vi "Get Default Trigger.vi"(7 "Trigger Direction":T2, 8 "error in (no error)":errorcluster, 11 "Item Ref in":T3 format="%.0x") -> (0 "error out":errorcluster, 2 "Default Trigger":T1, 3 "Item Ref out":T3 format="%.0x")   [LabVIEW 2015, in "Waveform Data Logger Shared.lvlib"]
uses:
  Waveform Data Logger Shared.lvlib
  <vilib>/NI Veristand/Custom Device API/Custom Device Item Ref.ctl
  Types/Trigger Direction.ctl
  Types/Default Trigger.ctl
  Globals/Property Strings.vi
  <vilib>/NI Veristand/Custom Device API/Get Item Property (Boolean).vi
  <vilib>/NI VeriStand/Custom Device API/Custom Device API.lvlib
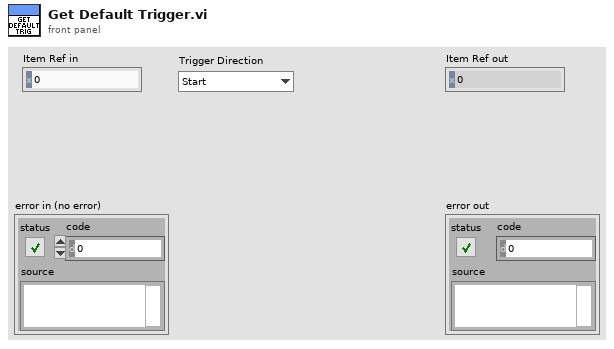
[diagram p1: front panel]
types:
  T1 = typedef "Waveform Data Logger Shared.lvlib/Default Trigger.ctl" = cluster{"Default State":bool}
  T2 = typedef "Waveform Data Logger Shared.lvlib/Trigger Direction.ctl" = enum16{"Start", "Stop"}
  T3 = typedef "Custom Device API.lvlib/Custom Device Item Ref.ctl" = u64
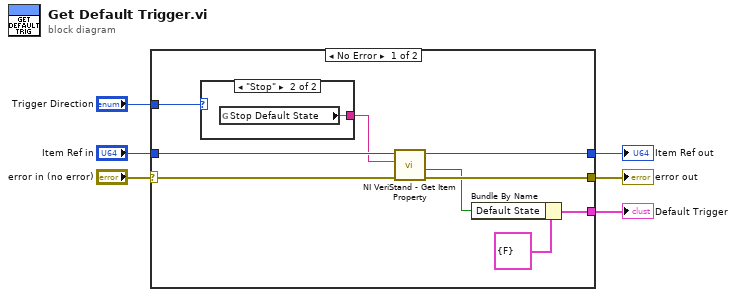
[diagram p0: block diagram]
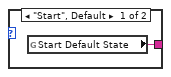
[diagram p2: hidden frame]
diagram:
  n1 = case shown="No Error" "error in (no error)" {
    selector: "error in (no error)" -> [w13 w18]
    tunnel: [w12 w19] -> w6
    tunnel: [w11 w18] -> w5
    tunnel: "Item Ref in" -> [w14 w19]
    tunnel: "Trigger Direction" -> [w15 _]
    tunnel: [w7 _] -> w1
    frame No Error {
      n2 = case shown="\"Stop\"" w15 {
        tunnel: [w16 w17] -> w10
        frame "Start", Default {
          n3 = global read "Property Strings.vi" "Start Default State"() -> (w16:string)
        }
        frame "Stop" {
          n4 = global read "Property Strings.vi" "Stop Default State"() -> (w17:string)
        }
      }
      n5 = call-poly <vilib>:"NI VeriStand - Get Item Property.vi"("error in (no error)"=w13, "Property Name"=w10, "Item Ref in"=w14) -> ("error out"=w11:errorcluster, "Value"=w8:bool, "Item Ref out"=w12:T3)  [unwired: 1 in, 5 out]
      n6 = Bundle By Name(cluster=T1 {"Default State"=FALSE} ("Default Trigger"), "Default State"=w8) -> (w7:T1)
    }
    frame Error {
    }
  }
  "Item Ref out" <- w6
  "error out" <- w5
  "Default Trigger" <- w1
